vi "Unpack Control Mouse Up.vi"(11 "ControlMouseUpMsg In":refnum<class "ControlMouseUpMsg.lvclass">) -> (0 "Button":u16, 1 "Coords":T2, 2 "Time":u32, 3 "Name":string, 4 "Mods":cluster{"Double Click":bool, "Menu Key":bool}, 6 "PlatMods":T1)   [LabVIEW 2015, in "ActorAutoRegistration.lvlib" / "ControlMouseUpMsg.lvclass"]
doc: "<License>\nCopyright © 2017 Composed Systems, LLC | All rights reserved\nwww.composed.io\n\nAuthor: Ethan Stern <ethan.stern@composed.io>\n\nThis software is provided \"AS IS\" WITHOUT WARRANTIES, either express or implied, AND IS FOR EDUCATIONAL PURPOSES ONLY.\n</License>"
uses:
  ControlMouseUpMsg.lvclass
  <vilib>/Utility/miscctls.llb/LVPoint32TypeDef.ctl
  ControlMouseUpMsg.lvclass/ControlMouseUpMsg.ctl
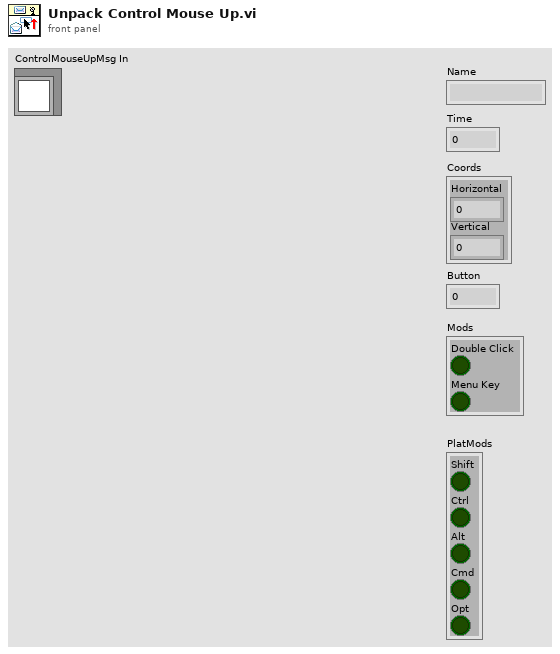
[diagram p1: front panel]
types:
  T1 = cluster{"Shift":bool, "Ctrl":bool, "Alt":bool, "Cmd":bool, "Opt":bool}
  T2 = typedef "LVPoint32TypeDef.ctl" = cluster{"Horizontal":i32, "Vertical":i32}
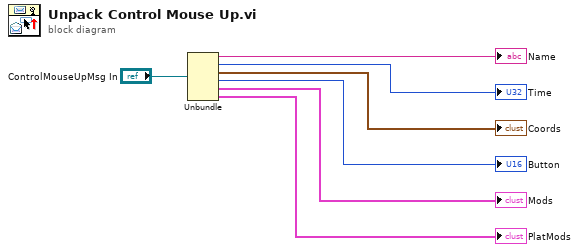
[diagram p0: block diagram]
diagram:
  n1 = Unbundle("ControlMouseUpMsg In") -> (→"Name":string, →"Time":u32, →"Coords":T2, →"Button":u16, →"Mods":cluster{"Double Click":bool, "Menu Key":bool}, →"PlatMods":T1)
